vi "filter data.vi"(8 "error in (no error)":errorcluster, 11 "LineCCD in":refnum<class "LineCCD.lvclass">=refnum) -> (0 "error out":errorcluster, 3 "LineCCD out":refnum<class "LineCCD.lvclass">)   [LabVIEW 2012, in "LineCCD.lvclass"]
uses:
  LineCCD.lvclass
  <vilib>/Distrio/LabbitMQ/2012/Connection/Connection_2012.lvclass
  <vilib>/Distrio/LabbitMQ/2012/Exchange/Exchange_2012.lvclass
  <vilib>/Distrio/LabbitMQ/2012/Queue/Queue_2012.lvclass
  <vilib>/Distrio/Murmex/ProceedMessage/ProceedMessage.lvclass
  <vilib>/Analysis/3filter.llb/Filter Passband Type.ctl
  LineCCD.lvclass/LineCCD.ctl
  <vilib>/Analysis/3filter.llb/Butterworth Filter (DBL).vi
  <vilib>/Analysis/NI_AALBase.lvlib
  <vilib>/Analysis/NI_AALPro.lvlib
panel:
  in  "low cutoff freq: fl 2":dbl=0.12500000000000006 format="%0.4f"
  in  "sampling freq: fs 2":dbl=1.0 format="%0.2f"
  in  "dt":dbl=0.01
  in  "low cutoff freq: fl":dbl=0.02 format="%0.4f"
  in  "high cutoff freq: fh":dbl=0.45 format="%0.2f"
  in  "sampling freq: fs":dbl=2.0 format="%0.2f"
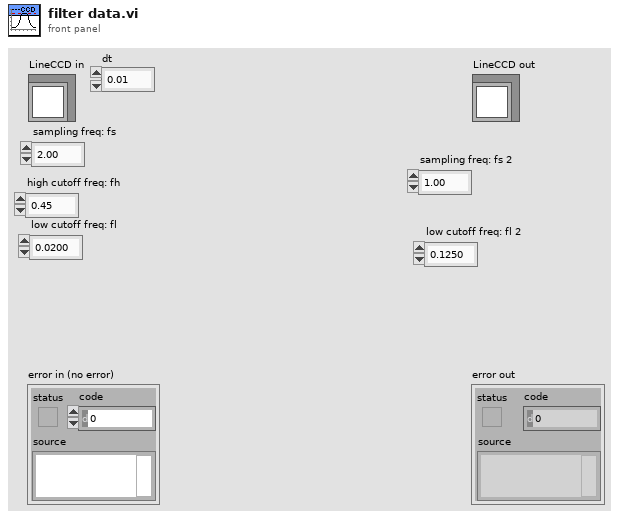
[diagram p1: front panel]
types:
  T1 = typedef "NI_AALBase.lvlib/Filter Passband Type.ctl" = enum32{"Lowpass", "Highpass", "Bandpass", "Bandstop"}
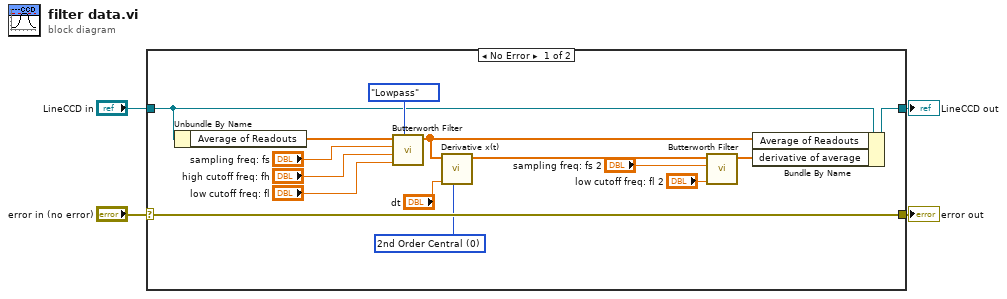
[diagram p0: block diagram]
diagram:
  n1 = case shown="No Error" "error in (no error)" {
    selector: "error in (no error)" -> [w19 w21]
    tunnel: [w19 w21] -> w3
    tunnel: [w12 w20] -> w1
    tunnel: "LineCCD in" -> [w13 w20]
    frame No Error {
      w10 = u16 0 items=["2nd Order Central", "4th Order Central", "Forward", "Backward"] ("method")
      n2 = Unbundle By Name(w13) -> ("Average of Readouts"=w18:dbl[])
      n3 = call-poly <vilib>:"Butterworth Filter.vi"("filter type"=Filter_Passband_Type."Lowpass", "low cutoff freq: fl"="low cutoff freq: fl", "high cutoff freq: fh"="high cutoff freq: fh", "sampling freq: fs"="sampling freq: fs", "X"=w18) -> ("Filtered X"=w11:dbl[])  [unwired: 3 in, 1 out]
      n4 = call <vilib>:"Derivative x(t).vi"("method"=w10, "dt"="dt", "X"=w11) -> ("dX/dt"=w8:dbl[])  [unwired: 7 in, 1 out]
      n5 = call-poly <vilib>:"Butterworth Filter.vi"("low cutoff freq: fl"="low cutoff freq: fl 2", "sampling freq: fs"="sampling freq: fs 2", "X"=w8) -> ("Filtered X"=w7:dbl[])  [unwired: 5 in, 1 out]
      n6 = Bundle By Name(cluster=w13, "Average of Readouts"=w11, "derivative of average"=w7) -> (w12:refnum<class "LineCCD.lvclass">)
    }
    frame Error {
    }
  }
  "error out" <- w3
  "LineCCD out" <- w1
